vi "TapeMonCountsCheck.vi"(8 "error in (no error)":errorcluster, 11 "TapeDrive in":refnum<class "TapeDrive.lvclass">) -> (0 "error out":errorcluster, 1 "MaxCountsOk":bool, 2 "maxCounts":dbl[](array[numeric]), 3 "TapeDrive out":refnum<class "TapeDrive.lvclass">)   [LabVIEW 2020, in "TapeDrive.lvclass"]
uses:
  TapeDrive.lvclass
  TapeDrive.lvclass/TapeDrive.ctl
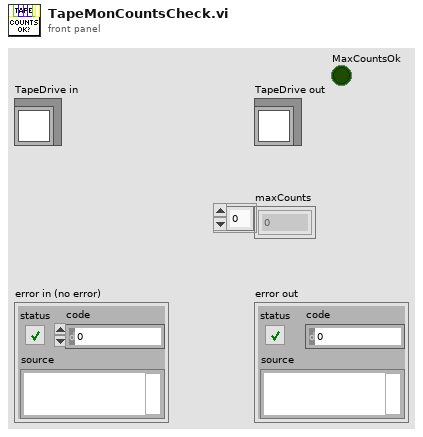
[diagram p1: front panel]
types:
  T1 = typedef "OnOffTypeDef.ctl" = enum16{"off", "on"}
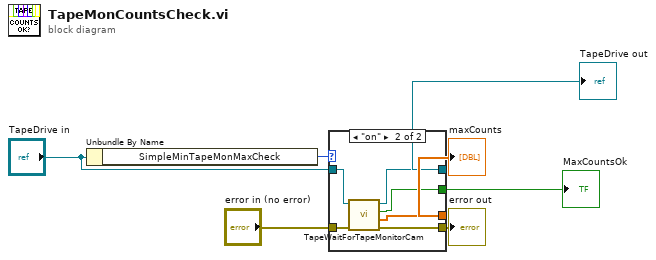
[diagram p0: block diagram]
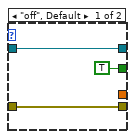
[diagram p2: hidden frame]
diagram:
  n1 = Unbundle By Name("TapeDrive in") -> ("SimpleMinTapeMonMaxCheck"=w4:T1)
  n2 = case shown="\"on\"" w4 {
    tunnel: "error in (no error)" -> [w9 w12]
    tunnel: "TapeDrive in" -> [w10 w16]
    tunnel: [w10 w15] -> w3
    tunnel: [_ w14] -> w5
    tunnel: [w9 w13] -> w6
    tunnel: [TRUE ("MaxCountsOk") w11] -> w1
    frame "off", Default {
    }
    frame "on" {
      n3 = call "TapeWaitForTapeMonitorCam.vi"("error in (no error)"=w12, "TapeDrive in"=w16) -> ("error out"=w13:errorcluster, "maxCounts"=w14:dbl[], "MaxCountsOk"=w11:bool, "TapeDrive out"=w15:refnum<class "TapeDrive.lvclass">)  [unwired: 6 in]
    }
  }
  "error out" <- w6
  "maxCounts" <- w5
  "TapeDrive out" <- w3
  "MaxCountsOk" <- w1
